vi "SNTP Light GUID Lookup.vi"() -> ()   [LabVIEW 2013, in "SNTP Light Custom Device Configuration.lvlib"]
doc: "Use this Global VI to access the GUIDs assigned to the page resources of the Custom Device."
uses:
  SNTP Light Custom Device Configuration.lvlib
panel:
  in  "Custom Device":string="523ce3d2-26a8-412b-8571-777b0d2adc68"
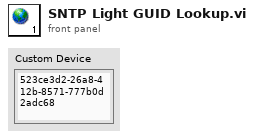
[diagram p1: front panel]
diagram:
